vi "nanocal -- nuclear schottky fit V7.vi"() -> ()   [LabVIEW 2021]
uses:
  filename-pattern.ctl
  show-win- control.ctl
  cursor winow.ctl
  nanocal_data_read_format.ctl
  3-lorentzian-parameters.ctl
  nameformattingitem.ctl
  nanocal_side_selector.ctl
  filename-action.ctl
  nanocal -- gradient descent -- parameters.ctl
  3-lorentzian-heat-response action.ctl
  nanocal-goodness-weighting-strategy.ctl
  nanocal generate curvature ellipse -- action.ctl
  3D curvature triplet control.ctl
  3D curvature tensor.ctl
  <vilib>/Analysis/Matrix/Datatypes/RealMatrix.ctl
  <vilib>/Analysis/Matrix/Datatypes/ComplexMatrix.ctl
  cursor window action.ctl
  cursor action.ctl
  2Dwindow.ctl
  publisher action.ctl
  <vilib>/Utility/miscctls.llb/LVMapReplaceAction.ctl
  mathematica string map action.ctl
  nanocal -- gradient descent -- action.ctl
  array action.ctl
  cursor sate.ctl
  nanocal -- defaut parameter manager action-- V1.ctl
  nanocal -- plotstring file action.ctl
  file -- read-write control.ctl
  array -- freq-voltage transformations action.ctl
  nanocal_raw_file_manage_action_V1.ctl
  KM_file -- read-write control.ctl
  replace cursor action stack.vi
  Q -- range multiplier -- real -- V2.vi
  Q - not nan and gtr than zero - Real.vi
  Q - not nan -- real.vi
  Q -- check range -- i -- real.vi
  array - smart min max.vi
  3-lorentzian-heat-response -- V4.vi/142dd4c5-f9ed-c64b-bc14-a88e3e2c450a.vi
  array -- bilinear regression 3D -- curvature wrapper -- V2.vi
  array -- gaussian random.vi
  <vilib>/Analysis/baseanly.llb/Mean.vi
  <vilib>/Analysis/baseanly.llb/Mean (DBL).vi
  <vilib>/AdvancedString/Delimited String to 1D String Array.vi
  array -- freq-voltage transformations.vi/05c44075-957c-bc42-b6fa-2799d0bc0485.vi
  tale of three indices.vi
  filter -- window span logic.vi
  linear interp iiii- complex - z-omega - divide.vi
  linear interpolation iiii- complex.vi
  containing bix.vi
  3D curvature tensor algebra --V2.vi
  array -- bilinear regression 3D -- V3.vi
  <vilib>/Array/Sort 2D Array - Pop Stack.vi
  <vilib>/Array/Sort 2D Array - Push Stack.vi
  array -- freq-voltage transformations.vi/05c44075-957c-bc42-b6fa-2799d0bc0485.vi/269d4b3b-47f5-49e3-8884-44851e4dd9d5.vi
  array -- freq-voltage transformations.vi/05c44075-957c-bc42-b6fa-2799d0bc0485.vi/6d99389c-673d-4efb-bf33-19b32bcf4cf8.vi
  command stack.vi
  tale of three indices -- check state.vi
  Q -- check range -- i -- integer.vi
  linear interp iiii- complex - z-omega.vi
  line -- complex.vi
  <vilib>/Analysis/7linalg.llb/Solve Linear Equations.vi
  <vilib>/Analysis/7linalg.llb/Solve Linear Equations (single right hand).vi
  array -- linear regression 3D -- V2.vi
  <vilib>/Analysis/baseanly.llb/A x B.vi
  <vilib>/Analysis/baseanly.llb/Real A x B.vi
  Q - not nan -- integer.vi
  <vilib>/Analysis/baseanly.llb/Complex A x B.vi
  <vilib>/Analysis/baseanly.llb/Solve Linear Equations By Cholesky.vi
  <vilib>/Analysis/baseanly.llb/Real Matrix to Compact Array.vi
  <vilib>/Analysis/baseanly.llb/Real Compact Tri-Matrix Linear Eqs.vi
  <vilib>/Analysis/Matrix/Numeric/Conversions/Array To Matrix.vi
  <vilib>/Analysis/Matrix/Numeric/Conversions/Array To Matrix - RA2.vi
  <vilib>/Analysis/7linalg.llb/Solve Linear Eqs (General).vi
  <vilib>/Analysis/7linalg.llb/Solve Linear Eqs (Gen, single right hand).vi
  <vilib>/Analysis/Matrix/Numeric/Conversions/Matrix To Array.vi
  <vilib>/Analysis/Matrix/Numeric/Conversions/Matrix To Array - RM.vi
  <vilib>/Analysis/7linalg.llb/Eigenvalues and Vectors.vi
  <vilib>/Analysis/7linalg.llb/Real Eigenvalues and Vectors.vi
  <vilib>/Analysis/baseanly.llb/Inverse Matrix.vi
  <vilib>/Analysis/baseanly.llb/Real Inverse Matrix.vi
  <vilib>/Analysis/polynomials.llb/Polynomial Roots.vi
  <vilib>/Analysis/polynomials.llb/Polynomial Roots (DBL).vi
  <vilib>/Comparison/Less/Less Functor/Less Functor.lvclass
  <vilib>/Analysis/Matrix/NI_Matrix.lvlib
panel:
  in  "tab 8":T1(tab)
  in  "sweeper panel":enum32{"main"}(tab)
  out "Plot: circles":cluster{"Freq out (Hz)":dbl[], dbl[]}[](graph)
  in  "scale gauge: Plot: circles":dbl(slide)=27302460.057190996 min=0.0 max=0.3 step=1e-06 scale=1000000.0..10000000000.0 scale format="%#_3p"
  in  "parameter tab":enum32{"logarithmic derivatives"}(tab)
  in  "factors":cluster{"scaling":dbl, "what":T2}[](array[cluster])=[{"scaling"=1.0, "what"=enum."ζ"}, {"scaling"=1.0, "what"=enum."τ1"}, {"scaling"=1.0, "what"=enum."τS"}, {"scaling"=1.0, "what"=enum."τN"}, {"scaling"=1.0, "what"=enum."τC"}, {"scaling"=1.0, "what"=enum."κ0"}]
  in  "tab77":enum32{"Page 1"}(tab)
  in  "τC":dbl(slide)=0.0015347438601793005 min=0.0 max=0.3 step=1e-06 scale=0.0001..1.0 scale format="%#_3p"
  in  "τN":dbl(slide)=0.020275054268168058 min=0.0 max=0.3 step=1e-06 scale=1e-06..1.0 scale format="%#_3p"
  in  "τS":dbl(slide)=0.018315346057340396 min=0.0 max=0.3 step=1e-06 scale=0.0001..1.0 scale format="%#_3p"
  in  "ζ":dbl(slide)=0.10152887026018578 min=0.0 max=0.3 step=1e-06 scale=1e-05..1.0 scale format="%#_3p"
  in  "T1":dbl(slide)=0.4652876432055127 min=0.0 max=0.3 step=1e-06 scale=0.0001..1.0 scale format="%#_3p"
  in  "κ0":dbl(slide)=1.5437103804183895e-09 min=0.0 max=0.3 step=1e-12 scale=1e-10..1e-06 scale format="%#_3p"
  in  "newton parameters":T3={"newton action"=enum."onlygrads", "weighting"=enum."dω √(|dz/dω|)", "PID-P"=9.612492635866019e-06, "PID-I"=12} {"PID-P" scale=1e-09..1.0 scale format="%#_3p"}
  out "vector v=dlogG/dlogα of logarithmic derivatives":dbl[](array[numeric])=[0.019124578634142967, 0.4891903036062691, -0.015428448808932498, -0.05822768648048974, -0.04691104340908931, 0.018178792884011388] format="%#11.9f"
  in  "tab 4":enum32{"Page 1"}(tab)
  in  "go / pause!":bool
  in  "plots tab":enum32{"Page 1"}(tab)
  in  "X selector":T2=enum."T (K)"
  out "Plot:  colors":cluster{"Freq out (Hz)":dbl[], dbl[]}[](graph)=[{"Freq out (Hz)"=[0.12, 0.148, 0.15, 0.17, 0.2, 0.25, 0.3, 0.36, 0.42, 0.52, 0.62, 0.82, 1.12, 1.7, 1.9, 3.1, 5.7], [0.62728998582, 0.2730109012575849, 0.4360358231158382, 0.31273882707493267, 0.21185679953244455, 0.14497429295634315, 0.10320507255338958, 0.06738649827292763, 0.022507492936216303, 0.021849716434935364, 0.021729475893381252, 0.0198519726342436, 0.016283381951146165, 0.01886089700009046, 0.017534515105553365, 0.01657901647493233, 0.017491792324152208]}, {"Freq out (Hz)"=[0.12, 0.148, 0.15, 0.17, 0.2, 0.25, 0.3, 0.36, 0.42, 0.52, 0.62, 0.82, 1.12, 1.7, 1.9, 3.1, 5.7], [0.23974349678, 0.07091543775458298, 0.13629832485566626, 0.15316677568416495, 0.17371303124805412, 0.27815367910908206, 0.4568771678095196, 0.03375938315839582, 0.03387143424300576, 0.033883152649051125, 0.03390178634313435, 0.03384656153160249, 0.03390452446017073, 0.03378369231014688, 0.02323861783817173, 0.029207680038740087, 0.02587551529326107]}, {"Freq out (Hz)"=[0.12, 0.148, 0.15, 0.17, 0.2, 0.25, 0.3, 0.36, 0.42, 0.52, 0.62, 0.82, 1.12, 1.7, 1.9, 3.1, 5.7], [0.076926495749, 0.13557684408337248, 0.03542880244691447, 0.02942840377205427, 0.02504707721851352, 0.020087180736490247, 0.018190810679879554, 0.0163524675075112, 0.016835987172777216, 0.01819702773822382, 0.020153498516221252, 0.023547995635674095, 0.031661688913314306, 0.03349591654527996, 0.014265591932458873, 0.009191722708188048, 0.005854448603805341]}, {"Freq out (Hz)"=[0.12, 0.148, 0.15, 0.17, 0.2, 0.25, 0.3, 0.36, 0.42, 0.52, 0.62, 0.82, 1.12, 1.7, 1.9, 3.1, 5.7], [0.159415903746, 0.04012911681217574, 0.042141009445427945, 0.032059842594624494, 0.02279985029361622, 0.018878235168909133, 0.020353539568818982, 5.5602042137039274e-05, 0.00021346840235837033, 0.00021340250099372794, 0.00021321792059620005, 0.00027413175252649695, 0.0002745370162211529, 0.0004261574975821111, 0.000383027800546881, 0.0002822141564676873, 0.00033678261197217014]}, {"Freq out (Hz)"=[0.12, 0.148, 0.15, 0.17, 0.2, 0.25, 0.3, 0.36, 0.42, 0.52, 0.62, 0.82, 1.12, 1.7, 1.9, 3.1, 5.7], [0.000763641667, 0.0009923872987074498, 0.0008634344957269274, 0.000966119229084584, 0.0011194877919145127, 0.0013606502621125451, 0.0015326336783234693, 0.002052818741953473, 0.0017781658353584764, 0.001801850307392029, 0.0018089734240976446, 0.002984103948241005, 0.003250738484609814, 0.0031602960429135524, 0.002949269667352954, 0.002421267656945163, 0.002022629565026247]}]
  in  "tab 55":enum32{"main", "more", "file", "notes"}(tab)
  in  "gradient descent monitor tab":enum32{"Page 2"}(tab)
  out "|dln G/dln α_i |":dbl(slide)=56.37329977448589 scale=0.001..1.0 scale format="%#_3p"
  out "Goodness":dbl(slide)=0.00019249505739334056 scale=0.001..1.0 scale format="%#_3p"
  in  "update rate":i32=1000
  in  "total # steps":i32=50000
  out "|v_i| = | dlogG/dlogα_i | (log scale slider)":dbl[](array[slide])=[0.019124578634142967, 0.4891903036062691, 0.015428448808932498, 0.05822768648048974, 0.04691104340908931, 0.018178792884011388] scale=1e-08..10.0 scale format="%#_2p"
  in  "oscillations & stuff tab":enum32{"Page 2", "Page 3"}(tab)
  in  "tab 9":enum32{"Page 1"}(tab)
  in  "#grad steps":i32=400
  out "Plot: oscillations":cluster{"Array":i32[], "Array":dbl[]}(graph)={"Array"=[0, 1, 2, 3, 4, 5, 6, 7, 8, 9, 10, 11, 12, 13, 14, 15, 16, 17, 18, 19, 20, 21, 22, 23, 24, 25, 26, 27, 28, 29, 30, 31, 32, 33, 34, 35, 36, 37, 38, 39, 40, 41, 42, 43, 44, 45, 46, 47, 48, 49, 50, 51, 52, 53, 54, 55, 56, 57, 58, 59, 60, 61, 62, 63, 64, 65, 66, 67, 68, 69, 70, 71, 72, 73, 74, 75, 76, 77, 78, 79, 80, 81, 82, 83, 84, 85, 86, 87, 88, 89, 90, 91, 92, 93, 94, 95, 96, 97, 98, 99, 100, 101, 102, 103, 104, 105, 106, 107, 108, 109, 110, 111, 112, 113, 114, 115, 116, 117, 118, 119, 120, 121, 122, 123, 124, 125, 126, 127, 128, 129, 130, 131, 132, 133, 134, 135, 136, 137, 138, 139, 140, 141, 142, 143, 144, 145, 146, 147, 148, 149, 150, 151, 152, 153, 154, 155, 156, 157, 158, 159, 160, 161, 162, 163, 164, 165, 166, 167, 168, 169, 170, 171, 172, 173, 174, 175, 176, 177, 178, 179, 180, 181, 182, 183, 184, 185, 186, 187, 188, 189, 190, 191, 192, 193, 194, 195, 196, 197, 198, 199, 200, 201, 202, 203, 204, 205, 206, 207, 208, 209, 210, 211, 212, 213, 214, 215, 216, 217, 218, 219, 220, 221, 222, 223, 224, 225, 226, 227, 228, 229, 230, 231, 232, 233, 234, 235, 236, 237, 238, 239, 240, 241, 242, 243, 244, 245, 246, 247, 248, 249, 250, 251, 252, 253, 254, 255, 256, 257, 258, 259, 260, 261, 262, 263, 264, 265, 266, 267, 268, 269, 270, 271, 272, 273, 274, 275, 276, 277, 278, 279, 280, 281, 282, 283, 284, 285, 286, 287, 288, 289, 290, 291, 292, 293, 294, 295, 296, 297, 298, 299, 300, 301, 302, 303, 304, 305, 306, 307, 308, 309, 310, 311, 312, 313, 314, 315, 316, 317, 318, 319, 320, 321, 322, 323, 324, 325, 326, 327, 328, 329, 330, 331, 332, 333, 334, 335, 336, 337, 338, 339, 340, 341, 342, 343, 344, 345, 346, 347, 348, 349, 350, 351, 352, 353, 354, 355, 356, 357, 358, 359, 360, 361, 362, 363, 364, 365, 366, 367, 368, 369, 370, 371, 372, 373, 374, 375, 376, 377, 378, 379, 380, 381, 382, 383, 384, 385, 386, 387, 388, 389, 390, 391, 392, 393, 394, 395, 396, 397, 398, 399], "Array"=[1.602606484205158e-10, 1.5784530103877918e-10, 1.554421775757514e-10, 1.5305127610697362e-10, 1.50672596713761e-10, 1.4830613717349908e-10, 1.4595189851617993e-10, 1.4360987835655876e-10, 1.4128007693858108e-10, 1.3896249247331328e-10, 1.366571244728644e-10, 1.3436397375038607e-10, 1.3208303678222122e-10, 1.2981431527598827e-10, 1.2755780643986664e-10, 1.2531351038227653e-10, 1.2308142688637752e-10, 1.2086155389218547e-10, 1.1865389137259534e-10, 1.1645843870419087e-10, 1.1427519523645076e-10, 1.1210415896360099e-10, 1.0994533143062965e-10, 1.0779870957466561e-10, 1.0566429301623811e-10, 1.0354208224323813e-10, 1.0143207495173605e-10, 9.933427143988746e-11, 9.724867078612053e-11, 9.517527174360274e-11, 9.311407274024096e-11, 9.106507570049403e-11, 8.902827753438577e-11, 8.700367854007178e-11, 8.499127760624482e-11, 8.299107321502186e-11, 8.100306582718882e-11, 7.902725476511933e-11, 7.706363748093831e-11, 7.511221524858329e-11, 7.317298530333874e-11, 7.124594973229384e-11, 6.933110642125435e-11, 6.74284519820885e-11, 6.55379904805544e-11, 6.365971733589791e-11, 6.179363292758977e-11, 5.99397377164159e-11, 5.809802901897594e-11, 5.62685072960558e-11, 5.445117121950782e-11, 5.2646021304328036e-11, 5.085305375580884e-11, 4.90722720976073e-11, 4.7303672887381507e-11, 4.554725501382424e-11, 4.380301939850735e-11, 4.2070964794598334e-11, 4.0351089955264693e-11, 3.864339363367393e-11, 3.6947876453242295e-11, 3.526453529688854e-11, 3.359337469115674e-11, 3.193438775136309e-11, 3.0287577648798955e-11, 2.8652942594530745e-11, 2.703048039304906e-11, 2.5420191342509502e-11, 2.3822075497122175e-11, 2.223613228768094e-11, 2.06623592205208e-11, 1.910075737984393e-11, 1.7551325329082448e-11, 1.6014061685878586e-11, 1.4488966911018267e-11, 1.2976039405303286e-11, 1.1475278301371905e-11, 9.986684249745428e-12, 8.510254865179076e-12, 7.045989171890893e-12, 5.593888741974029e-12, 4.153951678074683e-12, 2.726176543624975e-12, 1.310563718095667e-12, -9.288921086307578e-14, -1.4841796953761477e-12, -2.8633126685634336e-12, -4.230285284394231e-12, -5.5851015002064686e-12, -6.927759283121074e-12, -8.25825985286549e-12, -9.576604646007597e-12, -1.0882793255971579e-11, -1.2176828799838682e-11, -1.3458708648418638e-11, -1.4728437138520137e-11, -1.5986011993318616e-11, -1.7231435923319507e-11, -1.8464707058274063e-11, -1.968582908446967e-11, -2.0894800999019317e-11, -2.209162483480208e-11, -2.3276299155250077e-11, -2.4448826887709177e-11, -2.560920716481764e-11, -2.6757440393151283e-11, -2.7893529933736838e-11, -2.901747386211545e-11, -3.012927385880049e-11, -3.1228928893799884e-11, -3.231644387312847e-11, -3.339181557128479e-11, -3.445504490984068e-11, -3.550613473482685e-11, -3.654508477519275e-11, -3.7571895356199037e-11, -3.8586568022833806e-11, -3.95891017993151e-11, -4.057949917930792e-11, -4.1557760054392046e-11, -4.252388499377362e-11, -4.3477875135864916e-11, -4.4419729748829476e-11, -4.534945205816876e-11, -4.626704019363402e-11, -4.717249700125596e-11, -4.8065821125781866e-11, -4.8947015196402e-11, -4.981607826443947e-11, -5.06730123898784e-11, -5.1517817654033946e-11, -5.235049438216677e-11, -5.3171043468743656e-11, -5.397946564560108e-11, -5.4775762945618103e-11, -5.555993173671746e-11, -5.633197817174647e-11, -5.709189975704014e-11, -5.783969784785119e-11, -5.857537347417167e-11, -5.929892650047633e-11, -6.001035749597129e-11, -6.070966803274971e-11, -6.139685976421991e-11, -6.207193025092698e-11, -6.273488347731393e-11, -6.338571738339661e-11, -6.402443448994509e-11, -6.465103563721604e-11, -6.526551906338093e-11, -6.586788788552102e-11, -6.645814234758178e-11, -6.703628272061377e-11, -6.760230924856246e-11, -6.815622225668852e-11, -6.869802364234574e-11, -6.92277144355262e-11, -6.974529431096922e-11, -7.02507637023557e-11, -7.074412377520295e-11, -7.122537425846044e-11, -7.169451759158306e-11, -7.215155358483542e-11, -7.259648229242764e-11, -7.302930525934781e-11, -7.345002235007066e-11, -7.385863573300053e-11, -7.425514394446449e-11, -7.463954836682031e-11, -7.501184951506402e-11, -7.537205018101623e-11, -7.572014854863827e-11, -7.605614570213234e-11, -7.638004324069664e-11, -7.669184132696148e-11, -7.699154020487237e-11, -7.727914093152641e-11, -7.755464391349942e-11, -7.78180500452582e-11, -7.806935818839046e-11, -7.830857354706663e-11, -7.853569248920944e-11, -7.875071693927774e-11, -7.895364817120908e-11, -7.914448623921357e-11, -7.932323081803055e-11, -7.948988564815754e-11, -7.964444780224865e-11, -7.978691999080932e-11, -7.991730213252439e-11, -8.003559487791516e-11, -8.014180044959608e-11, -8.023591646232238e-11, -8.031794657527638e-11, -8.038788943320538e-11, -8.044574601189132e-11, -8.04915181544779e-11, -8.05252047496579e-11, -8.054680820978113e-11, -8.055632696275447e-11, -8.055376434249958e-11, -8.053911874981827e-11, -8.051239194653906e-11, -8.04735845560782e-11, -8.042269622606998e-11, -8.035972858281767e-11, -8.028468235815774e-11, -8.019755785024577e-11, -8.009835560118285e-11, -7.998707509597296e-11, -7.986372002090347e-11, -7.972828809914984e-11, -7.95807809028052e-11, -7.942120070869411e-11, -7.924954545683247e-11, -7.906581574353144e-11, -7.887001520086832e-11, -7.866214087439219e-11, -7.844219772432798e-11, -7.821018173912765e-11, -7.796609717428474e-11, -7.770994202402522e-11, -7.744171880911914e-11, -7.716142739404123e-11, -7.686906783300161e-11, -7.656464180651364e-11, -7.624814833879535e-11, -7.591959041140274e-11, -7.557896696723868e-11, -7.522627854840425e-11, -7.486152688962293e-11, -7.448471161142396e-11, -7.40958333372236e-11, -7.369489445226661e-11, -7.328189311340931e-11, -7.285683116379539e-11, -7.241971009420284e-11, -7.197052830543345e-11, -7.150928845378254e-11, -7.103598988872882e-11, -7.055063353184413e-11, -7.005321981680933e-11, -6.954375115597426e-11, -6.902222632961148e-11, -6.848864482272496e-11, -6.794301021318186e-11, -6.738532046810311e-11, -6.68155786774649e-11, -6.623378291680838e-11, -6.563993576111371e-11, -6.503403691222528e-11, -6.441608715618968e-11, -6.378608798378489e-11, -6.314403874448961e-11, -6.248993911304318e-11, -6.182379337204419e-11, -6.114559734731427e-11, -6.045535664959967e-11, -5.975306756550794e-11, -5.903873283264957e-11, -5.831235356233179e-11, -5.7573928372196825e-11, -5.682345953906924e-11, -5.606094722557936e-11, -5.5286391919618164e-11, -5.44997939464463e-11, -5.3701154769736706e-11, -5.289047322397204e-11, -5.2067752290708286e-11, -5.123299126521402e-11, -5.038619177379251e-11, -4.9527352867766855e-11, -4.8656474845292647e-11, -4.777355960372369e-11, -4.6878609040413785e-11, -4.597161998407158e-11, -4.5052597665972555e-11, -4.4121538020358564e-11, -4.317844546535346e-11, -4.222331826623377e-11, -4.125615745299155e-11, -4.027696354062284e-11, -3.928573888726736e-11, -3.828248259845832e-11, -3.726719502656142e-11, -3.623987665946765e-11, -3.520052871690445e-11, -3.414915171386784e-11, -3.308574705982066e-11, -3.2010313562140513e-11, -3.092285273871044e-11, -2.982336594478316e-11, -2.871185255694242e-11, -2.7588313442549958e-11, -2.6452750038173656e-11, -2.5305161340926502e-11, -2.414554913974208e-11, -2.297391384119621e-11, -2.1790256637911273e-11, -2.0594575659638528e-11, -1.9386874484245142e-11, -1.8167153220151333e-11, -1.6935410756049873e-11, -1.569164926034511e-11, -1.4435867459099486e-11, -1.3168069553596423e-11, -1.1888251315447448e-11, -1.0596416783305654e-11, -9.292566011381148e-12, -7.976699487564909e-12, -6.6488159379193834e-12, -5.3089191571521754e-12, -3.957007220804429e-12, -2.5930814570238048e-12, -1.2171420826507379e-12, 1.7080892364580713e-13, 1.5707728900134915e-12, 2.982747539627753e-12, 4.406732953803755e-12, 5.842729945693126e-12, 7.290735100059023e-12, 8.750749202948022e-12, 1.0222772254360121e-11, 1.1706803874824562e-11, 1.3202842438038084e-11, 1.4710886453222702e-11, 1.623093808878276e-11, 1.776299498657853e-11, 1.930705728213529e-11, 2.0863122400472875e-11, 2.2431192862361338e-11, 2.401126641808117e-11, 2.560334192922009e-11, 2.7207420181824676e-11, 2.8823499549591666e-11, 3.045157997831095e-11, 3.2091660709041014e-11, 3.3743741389416146e-11, 3.540782185680602e-11, 3.708389991570124e-11, 3.8771977083984846e-11, 4.047205078667668e-11, 4.218412199955869e-11, 4.390818950290344e-11, 4.564425335092104e-11, 4.7392310236794855e-11, 4.915236406365271e-11, 5.092441044047581e-11, 5.270845140014323e-11, 5.4504485722927515e-11, 5.631251069832324e-11, 5.813252732921742e-11, 5.996453756717396e-11, 6.18085360453921e-11, 6.366452509490653e-11, 6.553250376704033e-11, 6.74124723599491e-11, 6.930442759392128e-11, 7.120837207104207e-11, 7.31243031079111e-11, 7.505222097557891e-11, 7.699212393932203e-11, 7.894401362544372e-11, 8.090788729633348e-11, 8.288374595487834e-11, 8.48715881645104e-11, 8.687141330181343e-11, 8.888322109573688e-11, 9.090701219680204e-11, 9.294278403002877e-11, 9.499053635147157e-11, 9.7050269432181e-11, 9.912198254032056e-11, 1.0120567421221735e-10, 1.0330134515260277e-10, 1.0540899416885442e-10, 1.0752862134228748e-10, 1.0966022496528352e-10, 1.1180380444153135e-10, 1.1395936147864938e-10, 1.1612689087246719e-10, 1.1830639790847038e-10, 1.2049787841248057e-10, 1.2270133284528369e-10, 1.249167597974169e-10, 1.2714415837441345e-10, 1.2938353104283325e-10, 1.3163487230035027e-10, 1.3389818778481583e-10, 1.3617347074707138e-10, 1.3846072511734982e-10, 1.407599478869901e-10, 1.4307113935414784e-10, 1.4539429903093204e-10, 1.4772942613129614e-10, 1.5007651962524807e-10, 1.5243558027172935e-10, 1.5480660625470134e-10, 1.5718959873968139e-10, 1.5958455485353372e-10]}
  out "current step ind":i32=926
  out "current  ind":i32=1
  out "correct temperature":dbl=1040.0 min=10.0 max=10000.0 step=10.0
  in  "generate empty string from filelist !":bool
  in  "toggle generate labview files":bool
  in  "data file formatting":T6=enum."raw nanocal"
  in  "save data":enum32{"save/read"}(tab)
  in  "Save to file :s":bool
  in  "Freq sweep name template":T7={"prefix"="RuCl3-rod", "group"="f"}
  in  "Save folder":path=path "/opt/data"
  in  "freq sweep file name":string="f013_RuCl3-rod_082821.dat"
  in  "side":T8=enum."ref"
  in  "string notes":string="\"T\"-> 0.225000,    \"ζ\"-> 0.006057  , \"τ1\"-> 0.011106  , \"τS\"-> 0.134857  , \"τN\"-> 0.000042  , \"τC\"-> 0.012982  , \"κ0\"-> 0.000000101776  , \"mm1\"-> 0.000071  , \"mm2\"-> 0.148631  , \"mm3\"-> 0.011103 "
  in  "load! :l":bool
  in  "Read from file":path=path "/opt/new/Dropbox/shared_AkashAndreas/paper-CeCoIn5/Original RAW data/Original RAW files (IDS0396 to IDS0xxx)/IDS0446_220528_RAW_cal_CeCoIn5_5th_051_6T_0deg__fSweep_0.30K_raw_.dat"
  in  "parse! :p":bool
  in  "String":string=" <|    \"ζ\" -> 0.101528870260   ,  \"τ1\" -> 0.465287643206   ,  \"τS\" -> 0.018315346057   ,  \"τN\" -> 0.020275054268   ,  \"τC\" -> 0.001534743860   ,  \"κ0\" -> 0.000000001544   ,  \"mm1\" -> 0.000132261454   ,  \"mm2\" -> 0.020546066419   ,  \"mm3\" -> 0.488652499266   ,  \"T\" -> 0.300000000000   ,  \"B\" -> 6.000000000000   ,  \"θ\" -> 0.000000000000   ,  \"Reoff\" -> 0.000000000000   ,  \"Imoff\" -> 0.000000000000   ,  \"στ1\" -> 0.000000000000   ,  \"στS\" -> 0.000000000000   ,  \"στN\" -> 0.000000000000    |> "
  in  "newton is active":bool
  out "file IDS":string="IDS0446_220528_RAW_cal_"
  out "notes":string="------------\n\n/opt/new/Dropbox/desktop_data/Indium-nanocal-cell12-June2021/labview-ready-files\nIndium_June2021_*_ark.dat\n\n---------------------\n/opt/new/Dropbox/shared_AkashAndreas/paper-CeCoIn5/labviewreadydata\nCeCoIn5_*_labview_.dat\n--------------------------------\n\n  48 ->   <| \"ζ\"->  0.219100303741  , \"τ1\"-> 0.028643012604  , \"τS\"-> 0.279362928811  , \"τN\"-> 0.246156444058  , \"τC\"-> 0.001272401549  , \"κ0\"-> 0.000000000760  , \"mm1\"-> 0.000227975653  , \"mm2\"-> 0.014929571562  , \"mm3\"-> 0.655418694024  , \"T\"->  0.148000000000  , \"B\"-> 12.000000000000  , \"θ\"-> 0.000000000000  |>   , \r49 ->   <| \"ζ\"->  0.172530402516  , \"τ1\"-> 0.028151242536  , \"τS\"-> 0.147833386881  , \"τN\"-> 0.151615465647  , \"τC\"-> 0.001078987959  , \"κ0\"-> 0.000000001040  , \"mm1\"-> 0.000157922197  , \"mm2\"-> 0.013374167913  , \"mm3\"-> 0.366811023972  , \"T\"->  0.179000000000  , \"B\"-> 12.000000000000  , \"θ\"-> 0.000000000000  |>   , \r50 ->   <| \"ζ\"->  0.133463068512  , \"τ1\"-> 0.025720252342  , \"τS\"-> 0.123146502099  , \"τN\"-> 0.097478248186  , \"τC\"-> 0.001335222055  , \"κ0\"-> 0.000000001204  , \"mm1\"-> 0.000155896243  , \"mm2\"-> 0.013755191011  , \"mm3\"-> 0.263214393590  , \"T\"->  0.197000000000  , \"B\"-> 12.000000000000  , \"θ\"-> 0.000000000000  |>   , \r51 ->   <| \"ζ\"->  0.081993362741  , \"τ1\"-> 0.028064095915  , \"τS\"-> 0.091433392476  , \"τN\"-> 0.030443971714  , \"τC\"-> 0.001450504959  , \"κ0\"-> 0.000000001536  , \"mm1\"-> 0.000108446090  , \"mm2\"-> 0.019905820843  , \"mm3\"-> 0.141370833064  , \"T\"->  0.250000000000  , \"B\"-> 12.000000000000  , \"θ\"-> 0.000000000000  |>   , \r52 ->   <| \"ζ\"->  0.054088186012  , \"τ1\"-> 0.023838802615  , \"τS\"-> 0.069079396629  , \"τN\"-> 0.016435267456  , \"τC\"-> 0.002025071743  , \"κ0\"-> 0.000000001955  , \"mm1\"-> 0.000101234646  , \"mm2\"-> 0.018244822177  , \"mm3\"-> 0.097657814678  , \"T\"->  0.300000000000  , \"B\"-> 12.000000000000  , \"θ\"-> 0.000000000000  |>   , \r53 ->   <| \"ζ\"->  0.039314966212  , \"τ1\"-> 0.020712803909  , \"τS\"-> 0.055413767550  , \"τN\"-> 0.008474403424  , \"τC\"-> 0.002674063387  , \"κ0\"-> 0.000000002415  , \"mm1\"-> 0.000096818147  , \"mm2\"-> 0.017190811405  , \"mm3\"-> 0.072499170001  , \"T\"->  0.360000000000  , \"B\"-> 12.000000000000  , \"θ\"-> 0.000000000000  |>   , \r54 ->   <| \"ζ\"->  0.031945976845  , \"τ1\"-> 0.019000922826  , \"τS\"-> 0.045624146388  , \"τN\"-> 0.005314716063  , \"τC\"-> 0.002488383471  , \"κ0\"-> 0.000000002954  , \"mm1\"-> 0.000073272643  , \"mm2\"-> 0.016306894362  , \"mm3\"-> 0.057675293464  , \"T\"->  0.430000000000  , \"B\"-> 12.000000000000  , \"θ\"-> 0.000000000000  |>   , \r55 ->   <| \"ζ\"->  0.023031239946  , \"τ1\"-> 0.018268814012  , \"τS\"-> 0.037269400776  , \"τN\"-> 0.002696792890  , \"τC\"-> 0.003257395394  , \"κ0\"-> 0.000000003720  , \"mm1\"-> 0.000067670174  , \"mm2\"-> 0.016445281937  , \"mm3\"-> 0.045899921957  , \"T\"->  0.512000000000  , \"B\"-> 12.000000000000  , \"θ\"-> 0.000000000000  |>   , \r56 ->   <| \"ζ\"->  0.019920170845  , \"τ1\"-> 0.016368892412  , \"τS\"-> 0.030579536580  , \"τN\"-> 0.001736017565  , \"τC\"-> 0.004971418152  , \"κ0\"-> 0.000000004410  , \"mm1\"-> 0.000083939556  , \"mm2\"-> 0.015095997595  , \"mm3\"-> 0.039119658918  , \"T\"->  0.610000000000  , \"B\"-> 12.000000000000  , \"θ\"-> 0.000000000000  |>   , \r57 ->   <| \"ζ\"->  0.017558473054  , \"τ1\"-> 0.014545104284  , \"τS\"-> 0.022979681288  , \"τN\"-> 0.000840829385  , \"τC\"-> 0.005228030240  , \"κ0\"-> 0.000000006068  , \"mm1\"-> 0.000073916527  , \"mm2\"-> 0.013750428362  , \"mm3\"-> 0.030187552103  , \"T\"->  0.810000000000  , \"B\"-> 12.000000000000  , \"θ\"-> 0.000000000000  |>   , \r58 ->   <| \"ζ\"->  0.011916480594  , \"τ1\"-> 0.012551282481  , \"τS\"-> 0.018233218660  , \"τN\"-> 0.000345702746  , \"τC\"-> 0.004699451527  , \"κ0\"-> 0.000000008451  , \"mm1\"-> 0.000044190864  , \"mm2\"-> 0.012162820727  , \"mm3\"-> 0.023844039179  , \"T\"->  1.120000000000  , \"B\"-> 12.000000000000  , \"θ\"-> 0.000000000000  |>   , \r59 ->   <| \"ζ\"->  0.012831327568  , \"τ1\"-> 0.013315909415  , \"τS\"-> 0.012590836847  , \"τN\"-> 0.000065003013  , \"τC\"-> 0.005276356243  , \"κ0\"-> 0.000000013610  , \"mm1\"-> 0.000047406274  , \"mm2\"-> 0.013137605540  , \"mm3\"-> 0.018225484932  , \"T\"->  1.800000000000  , \"B\"-> 12.000000000000  , \"θ\"-> 0.000000000000  |>   , \r60 ->   <| \"ζ\"->  0.019774146838  , \"τ1\"-> 0.013257273421  , \"τS\"-> 0.007064131508  , \"τN\"-> 0.000028000819  , \"τC\"-> 0.006942241845  , \"κ0\"-> 0.000000023477  , \"mm1\"-> 0.000068886863  , \"mm2\"-> 0.012935419574  , \"mm3\"-> 0.014427582022  , \"T\"->  3.000000000000  , \"B\"-> 12.000000000000  , \"θ\"-> 0.000000000000  |>   , \r61 ->   <| \"ζ\"->  0.029251354442  , \"τ1\"-> 0.014634751206  , \"τS\"-> 0.003873958746  , \"τN\"-> 0.000007000487  , \"τC\"-> 0.006827504775  , \"κ0\"-> 0.000000056438  , \"mm1\"-> 0.000072018576  , \"mm2\"-> 0.010723236476  , \"mm3\"-> 0.014661483476  , \"T\"->  5.500000000000  , \"B\"-> 12.000000000000  , \"θ\"-> 0.000000000000  |>   , \r70 ->   <| \"ζ\"->  0.166131699293  , \"τ1\"-> 0.072775930308  , \"τS\"-> 0.042465819987  , \"τN\"-> 0.161702990281  , \"τC\"-> 0.001278548133  , \"κ0\"-> 0.000000001029  , \"mm1\"-> 0.000178150965  , \"mm2\"-> 0.012296129795  , \"mm3\"-> 0.299667919341  , \"T\"->  0.179000000000  , \"B\"-> 12.000000000000  , \"θ\"-> 90.000000000000  |>   , \r71 ->   <| \"ζ\"->  0.300863384227  , \"τ1\"-> 0.104924004009  , \"τS\"-> 0.071070599729  , \"τN\"-> 0.992887187112  , \"τC\"-> 0.001721587800  , \"κ0\"-> 0.000000000548  , \"mm1\"-> 0.000392216822  , \"mm2\"-> 0.006637384427  , \"mm3\"-> 1.483679717825  , \"T\"->  0.120000000000  , \"B\"-> 12.000000000000  , \"θ\"-> 90.000000000000  |>   , \r72 ->   <| \"ζ\"->  0.222191124978  , \"τ1\"-> 0.096157808510  , \"τS\"-> 0.068016409177  , \"τN\"-> 0.365932480375  , \"τC\"-> 0.001342124138  , \"κ0\"-> 0.000000000769  , \"mm1\"-> 0.000240761160  , \"mm2\"-> 0.013184061080  , \"mm3\"-> 0.614443591912  , \"T\"->  0.148000000000  , \"B\"-> 12.000000000000  , \"θ\"-> 90.000000000000  |>   , \r73 ->   <| \"ζ\"->  0.136299067728  , \"τ1\"-> 0.070555788073  , \"τS\"-> 0.041728112583  , \"τN\"-> 0.122673380524  , \"τC\"-> 0.001576035942  , \"κ0\"-> 0.000000001215  , \"mm1\"-> 0.000183611814  , \"mm2\"-> 0.014077355758  , \"mm3\"-> 0.244680119794  , \"T\"->  0.197000000000  , \"B\"-> 12.000000000000  , \"θ\"-> 90.000000000000  |>   , \r74 ->   <| \"ζ\"->  0.083818989463  , \"τ1\"-> 0.054019568165  , \"τS\"-> 0.033709166928  , \"τN\"-> 0.048192327645  , \"τC\"-> 0.001574712191  , \"κ0\"-> 0.000000001532  , \"mm1\"-> 0.000117096712  , \"mm2\"-> 0.016005996433  , \"mm3\"-> 0.128237582295  , \"T\"->  0.249000000000  , \"B\"-> 12.000000000000  , \"θ\"-> 90.000000000000  |>   , \r75 ->   <| \"ζ\"->  0.057938569833  , \"τ1\"-> 0.045244527663  , \"τS\"-> 0.029709028064  , \"τN\"-> 0.023577376257  , \"τC\"-> 0.002006607539  , \"κ0\"-> 0.000000001948  , \"mm1\"-> 0.000103608352  , \"mm2\"-> 0.017542867394  , \"mm3\"-> 0.085978401835  , \"T\"->  0.300000000000  , \"B\"-> 12.000000000000  , \"θ\"-> 90.000000000000  |>   , \r76 ->   <| \"ζ\"->  0.044154556051  , \"τ1\"-> 0.038823125235  , \"τS\"-> 0.027069314930  , \"τN\"-> 0.013601990730  , \"τC\"-> 0.002287979276  , \"κ0\"-> 0.000000002359  , \"mm1\"-> 0.000089763345  , \"mm2\"-> 0.018083678254  , \"mm3\"-> 0.065404792018  , \"T\"->  0.360000000000  , \"B\"-> 12.000000000000  , \"θ\"-> 90.000000000000  |>   , \r77 ->   <| \"ζ\"->  0.032748569996  , \"τ1\"-> 0.031072007290  , \"τS\"-> 0.024343937548  , \"τN\"-> 0.006961654481  , \"τC\"-> 0.002967111565  , \"κ0\"-> 0.000000002964  , \"mm1\"-> 0.000084402249  , \"mm2\"-> 0.018055855929  , \"mm3\"-> 0.048229666078  , \"T\"->  0.430000000000  , \"B\"-> 12.000000000000  , \"θ\"-> 90.000000000000  |>   , \r78 ->   <| \"ζ\"->  0.027599263457  , \"τ1\"-> 0.026239105728  , \"τS\"-> 0.022370859308  , \"τN\"-> 0.003857632966  , \"τC\"-> 0.003499360499  , \"κ0\"-> 0.000000003681  , \"mm1\"-> 0.000081816106  , \"mm2\"-> 0.017901054668  , \"mm3\"-> 0.038707974796  , \"T\"->  0.512000000000  , \"B\"-> 12.000000000000  , \"θ\"-> 90.000000000000  |>   , \r79 ->   <| \"ζ\"->  0.020568815513  , \"τ1\"-> 0.023045965648  , \"τS\"-> 0.020791387386  , \"τN\"-> 0.002229171297  , \"τC\"-> 0.004427475438  , \"κ0\"-> 0.000000004398  , \"mm1\"-> 0.000074037290  , \"mm2\"-> 0.017820522459  , \"mm3\"-> 0.033072945644  , \"T\"->  0.610000000000  , \"B\"-> 12.000000000000  , \"θ\"-> 90.000000000000  |>   , \r80 ->   <| \"ζ\"->  0.016159836955  , \"τ1\"-> 0.019958638777  , \"τS\"-> 0.018730096307  , \"τN\"-> 0.000899236968  , \"τC\"-> 0.005152267403  , \"κ0\"-> 0.000000006087  , \"mm1\"-> 0.000064651231  , \"mm2\"-> 0.017530317649  , \"mm3\"-> 0.027462477400  , \"T\"->  0.810000000000  , \"B\"-> 12.000000000000  , \"θ\"-> 90.000000000000  |>   , \r81 ->   <| \"ζ\"->  0.014495870556  , \"τ1\"-> 0.019990087457  , \"τS\"-> 0.016832201384  , \"τN\"-> 0.000455517238  , \"τC\"-> 0.005555782498  , \"κ0\"-> 0.000000008420  , \"mm1\"-> 0.000060055560  , \"mm2\"-> 0.018114231010  , \"mm3\"-> 0.024909902538  , \"T\"->  1.100000000000  , \"B\"-> 12.000000000000  , \"θ\"-> 90.000000000000  |>   , \r82 ->   <| \"ζ\"->  0.014043763709  , \"τ1\"-> 0.018292068543  , \"τS\"-> 0.011311396743  , \"τN\"-> 0.000128802259  , \"τC\"-> 0.008087849636  , \"κ0\"-> 0.000000014258  , \"mm1\"-> 0.000065912054  , \"mm2\"-> 0.017276417784  , \"mm3\"-> 0.020638450794  , \"T\"->  1.800000000000  , \"B\"-> 12.000000000000  , \"θ\"-> 90.000000000000  |>   , \r83 ->   <| \"ζ\"->  0.016187684631  , \"τ1\"-> 0.018325345271  , \"τS\"-> 0.007510087776  , \"τN\"-> 0.000028419157  , \"τC\"-> 0.008115463080  , \"κ0\"-> 0.000000024747  , \"mm1\"-> 0.000062903858  , \"mm2\"-> 0.015524812312  , \"mm3\"-> 0.018513630087  , \"T\"->  3.000000000000  , \"B\"-> 12.000000000000  , \"θ\"-> 90.000000000000  |>   , \r84 ->   <| \"ζ\"->  0.027897403691  , \"τ1\"-> 0.014639690770  , \"τS\"-> 0.004105291179  , \"τN\"-> 0.000006999171  , \"τC\"-> 0.007414449545  , \"κ0\"-> 0.000000059701  , \"mm1\"-> 0.000073450671  , \"mm2\"-> 0.011534391407  , \"mm3\"-> 0.014673310811  , \"T\"->  5.700000000000  , \"B\"-> 12.000000000000  , \"θ\"-> 90.000000000000  |>   , \r"
  in  "backup string :b":string=" <| \"ζ\"->  0.167234158379  , \"τ1\"-> 0.020665214756  , \"τS\"-> 0.072250691270  , \"τN\"-> 0.020708769022  , \"τC\"-> 0.001243822553  , \"κ0\"-> 0.000000001059  , \"mm1\"-> 0.000000000000  , \"mm2\"-> 0.000000000000  , \"mm3\"-> 0.000000000000  , \"T\"->  5.700000000000  , \"B\"-> 12.000000000000  , \"θ\"-> 45.000000000000  |> "
  in  "tab 7":enum32{"Page 1"}(tab)
  in  "tab 3":enum32{"Page 1"}(tab)
  out "key":string="IDS0446_220528_RAW_cal__ref_"
  out "T (K)":dbl=0.3 format="%#_10f"
  out "θ (deg)":dbl format="%#_10f"
  out "B (T)":dbl=6.0
  in  "tab 6":enum32{"Page 1"}(tab)
  in  "τ→Math! :p":bool
  in  "selection :|\\":u16(ring)=6 caption="files" items=["IDS063_210603_RAW_cal_Indium_2nd_063_C(f)_35.0T_0.8K_0deg_Tdep_dc_bias_raw_.dat", "IDS008_210601_RAW_cal_Indium_2nd_008_C(f)_35.0T_1.0K_0deg_Bdep_raw_.dat", "IDS013_210601_RAW_cal_Indium_2nd_013_C(f)_35.0T_1.0K_0deg_Bdep_raw_.dat", "IDS061_210603_RAW_cal_Indium_2nd_061_C(f)_35.0T_1.0K_0deg_Tdep_dc_bias_raw_.dat", "IDS076_210604_RAW_cal_Indium_2nd_076_C(f)_35.0T_1.2K_0deg_Tdep_dc_bias_raw_.dat", "IDS064_210603_RAW_cal_Indium_2nd_064_C(f)_35.0T_1.38K_0deg_Tdep_dc_bias_raw_.dat", "IDS075_210604_RAW_cal_Indium_2nd_075_C(f)_35.0T_1.6K_0deg_Tdep_dc_bias_raw_.dat", "IDS065_210603_RAW_cal_Indium_2nd_065_C(f)_35.0T_1.83K_0deg_Tdep_dc_bias_raw_.dat", "IDS074_210604_RAW_cal_Indium_2nd_074_C(f)_35.0T_2.13K_0deg_Tdep_dc_bias_raw_.dat", "IDS066_210603_RAW_cal_Indium_2nd_066_C(f)_35.0T_2.55K_0deg_Tdep_dc_bias_raw_.dat", "IDS019_210602_RAW_cal_Indium_2nd_019_C(f)_35.0T_3.0K_0deg_Tdep_raw_.dat", "IDS069_210604_RAW_cal_Indium_2nd_069_C(f)_35.0T_4.0K_0deg_Tdep_dc_bias_raw_.dat", "IDS067_210603_RAW_cal_Indium_2nd_067_C(f)_35.0T_8.2K_0deg_Tdep_dc_bias_raw_.dat"]
  in  "tab 5":enum32{"Page 1"}(tab)
  in  "Math→τ! :q":bool
  in  "tab 44":enum32{"default values "}(tab)
  in  "defaults selector":T9(array[cluster])=[{"Plost: sweep window"=enum."ζ", "used default"=FALSE}, {"Plost: sweep window"=enum."τ1", "used default"=FALSE}, {"Plost: sweep window"=enum."τS", "used default"=FALSE}, {"Plost: sweep window"=enum."τN", "used default"=FALSE}, {"Plost: sweep window"=enum."τC", "used default"=FALSE}, {"Plost: sweep window"=enum."κ0", "used default"=FALSE}]
  in  "default values string":string="\"0\"->   <|\"T\" -> 0.120000, \"τN\"-> 0.670097, \"τC\"-> 0.003, \"ζ\"-> 0.368640, \"κ0\"-> 0.00000000044100|>   ,\n\"1\"->   <|\"T\" -> 0.220000, \"τN\"-> 0.057428, \"τC\"-> 0.001386, \"ζ\"-> 0.131633, \"κ0\"-> 0.00000000120283|>   ,\n\"2\"->   <|\"T\" -> 0.320000, \"τN\"-> 0.014576, \"τC\"-> 0.001971, \"ζ\"-> 0.063259, \"κ0\"-> 0.00000000186767|>   ,\n\"3\"->   <|\"T\" -> 0.420000, \"τN\"-> 0.005816, \"τC\"-> 0.002645, \"ζ\"-> 0.041943, \"κ0\"-> 0.00000000259214|>   ,\n\"4\"->   <|\"T\" -> 0.520000, \"τN\"-> 0.002807, \"τC\"-> 0.003188, \"ζ\"-> 0.030182, \"κ0\"-> 0.00000000339327|>   ,\n\"5\"->   <|\"T\" -> 0.620000, \"τN\"-> 0.001928, \"τC\"-> 0.003634, \"ζ\"-> 0.025126, \"κ0\"-> 0.00000000404950|>   ,\n\"6\"->   <|\"T\" -> 0.720000, \"τN\"-> 0.001251, \"τC\"-> 0.004021, \"ζ\"-> 0.023386, \"κ0\"-> 0.00000000484450|>   ,\n\"7\"->   <|\"T\" -> 0.820000, \"τN\"-> 0.000866, \"τC\"-> 0.004389, \"ζ\"-> 0.022054, \"κ0\"-> 0.00000000563624|>   ,\n\"8\"->   <|\"T\" -> 0.920000, \"τN\"-> 0.000673, \"τC\"-> 0.004723, \"ζ\"-> 0.021623, \"κ0\"-> 0.00000000639866|>   ,\n\"9\"->   <|\"T\" -> 1.020000, \"τN\"-> 0.000537, \"τC\"-> 0.005044, \"ζ\"-> 0.021243, \"κ0\"-> 0.00000000716107|>   ,\n\"10\"->   <|\"T\" -> 1.120000, \"τN\"-> 0.000431, \"τC\"-> 0.005344, \"ζ\"-> 0.020967, \"κ0\"-> 0.00000000793323|>   ,\n\"11\"->   <|\"T\" -> 1.220000, \"τN\"-> 0.000336, \"τC\"-> 0.005596, \"ζ\"-> 0.020955, \"κ0\"-> 0.00000000874437|>   ,\n\"12\"->   <|\"T\" -> 1.320000, \"τN\"-> 0.000267, \"τC\"-> 0.005838, \"ζ\"-> 0.020944, \"κ0\"-> 0.00000000955551|>   ,\n\"13\"->   <|\"T\" -> 1.420000, \"τN\"-> 0.000216, \"τC\"-> 0.006071, \"ζ\"-> 0.020934, \"κ0\"-> 0.00000001036666|>   ,\n\"14\"->   <|\"T\" -> 1.520000, \"τN\"-> 0.000177, \"τC\"-> 0.006297, \"ζ\"-> 0.020925, \"κ0\"-> 0.00000001117780|>   ,\n\"15\"->   <|\"T\" -> 1.620000, \"τN\"-> 0.000147, \"τC\"-> 0.006517, \"ζ\"-> 0.020916, \"κ0\"-> 0.00000001198894|>   ,\n\"16\"->   <|\"T\" -> 1.720000, \"τN\"-> 0.000123, \"τC\"-> 0.006730, \"ζ\"-> 0.020907, \"κ0\"-> 0.00000001280009|>   ,\n\"17\"->   <|\"T\" -> 1.820000, \"τN\"-> 0.000105, \"τC\"-> 0.006885, \"ζ\"-> 0.020876, \"κ0\"-> 0.00000001362415|>   ,\n\"18\"->   <|\"T\" -> 1.920000, \"τN\"-> 0.000091, \"τC\"-> 0.006831, \"ζ\"-> 0.020754, \"κ0\"-> 0.00000001449990|>   ,\n\"19\"->   <|\"T\" -> 2.020000, \"τN\"-> 0.000080, \"τC\"-> 0.006781, \"ζ\"-> 0.020639, \"κ0\"-> 0.00000001537565|>   ,\n\"20\"->   <|\"T\" -> 2.120000, \"τN\"-> 0.000070, \"τC\"-> 0.006733, \"ζ\"-> 0.020530, \"κ0\"-> 0.00000001625140|>   ,\n\"21\"->   <|\"T\" -> 2.220000, \"τN\"-> 0.000062, \"τC\"-> 0.006687, \"ζ\"-> 0.020427, \"κ0\"-> 0.00000001712715|>   ,\n\"22\"->   <|\"T\" -> 2.320000, \"τN\"-> 0.000056, \"τC\"-> 0.006644, \"ζ\"-> 0.020329, \"κ0\"-> 0.00000001800290|>   ,\n\"23\"->   <|\"T\" -> 2.420000, \"τN\"-> 0.000050, \"τC\"-> 0.006603, \"ζ\"-> 0.020235, \"κ0\"-> 0.00000001887865|>   ,\n\"24\"->   <|\"T\" -> 2.520000, \"τN\"-> 0.000045, \"τC\"-> 0.006564, \"ζ\"-> 0.020146, \"κ0\"-> 0.00000001975440|>   ,\n\"25\"->   <|\"T\" -> 2.620000, \"τN\"-> 0.000040, \"τC\"-> 0.006527, \"ζ\"-> 0.020060, \"κ0\"-> 0.00000002063015|>   ,\n\"26\"->   <|\"T\" -> 2.720000, \"τN\"-> 0.000037, \"τC\"-> 0.006491, \"ζ\"-> 0.019978, \"κ0\"-> 0.00000002150590|>   ,\n\"27\"->   <|\"T\" -> 2.820000, \"τN\"-> 0.000033, \"τC\"-> 0.006457, \"ζ\"-> 0.019899, \"κ0\"-> 0.00000002238165|>   ,\n\"28\"->   <|\"T\" -> 2.920000, \"τN\"-> 0.000030, \"τC\"-> 0.006424, \"ζ\"-> 0.019824, \"κ0\"-> 0.00000002325740|>   ,\n\"29\"->   <|\"T\" -> 3.020000, \"τN\"-> 0.000028, \"τC\"-> 0.006374, \"ζ\"-> 0.019852, \"κ0\"-> 0.00000002421662|>   ,\n\"30\"->   <|\"T\" -> 3.120000, \"τN\"-> 0.000026, \"τC\"-> 0.006255, \"ζ\"-> 0.020282, \"κ0\"-> 0.00000002550973|>   ,\n\"31\"->   <|\"T\" -> 3.220000, \"τN\"-> 0.000024, \"τC\"-> 0.006143, \"ζ\"-> 0.020708, \"κ0\"-> 0.00000002680284|>   ,\n\"32\"->   <|\"T\" -> 3.320000, \"τN\"-> 0.000023, \"τC\"-> 0.006036, \"ζ\"-> 0.021130, \"κ0\"-> 0.00000002809596|>   ,\n\"33\"->   <|\"T\" -> 3.420000, \"τN\"-> 0.000021, \"τC\"-> 0.005933, \"ζ\"-> 0.021547, \"κ0\"-> 0.00000002938907|>   ,\n\"34\"->   <|\"T\" -> 3.520000, \"τN\"-> 0.000020, \"τC\"-> 0.005836, \"ζ\"-> 0.021960, \"κ0\"-> 0.00000003068218|>   ,\n\"35\"->   <|\"T\" -> 3.620000, \"τN\"-> 0.000019, \"τC\"-> 0.005742, \"ζ\"-> 0.022368, \"κ0\"-> 0.00000003197529|>   ,\n\"36\"->   <|\"T\" -> 3.720000, \"τN\"-> 0.000018, \"τC\"-> 0.005653, \"ζ\"-> 0.022774, \"κ0\"-> 0.00000003326840|>   ,\n\"37\"->   <|\"T\" -> 3.820000, \"τN\"-> 0.000017, \"τC\"-> 0.005567, \"ζ\"-> 0.023175, \"κ0\"-> 0.00000003456151|>   ,\n\"38\"->   <|\"T\" -> 3.920000, \"τN\"-> 0.000016, \"τC\"-> 0.005485, \"ζ\"-> 0.023573, \"κ0\"-> 0.00000003585462|>   ,\n\"39\"->   <|\"T\" -> 4.020000, \"τN\"-> 0.000015, \"τC\"-> 0.005406, \"ζ\"-> 0.023967, \"κ0\"-> 0.00000003714773|>   ,\n\"40\"->   <|\"T\" -> 4.120000, \"τN\"-> 0.000014, \"τC\"-> 0.005330, \"ζ\"-> 0.024358, \"κ0\"-> 0.00000003844084|>   ,\n\"41\"->   <|\"T\" -> 4.220000, \"τN\"-> 0.000013, \"τC\"-> 0.005257, \"ζ\"-> 0.024746, \"κ0\"-> 0.00000003973396|>   ,\n\"42\"->   <|\"T\" -> 4.320000, \"τN\"-> 0.000013, \"τC\"-> 0.005186, \"ζ\"-> 0.025131, \"κ0\"-> 0.00000004102707|>   ,\n\"43\"->   <|\"T\" -> 4.420000, \"τN\"-> 0.000012, \"τC\"-> 0.005118, \"ζ\"-> 0.025512, \"κ0\"-> 0.00000004232018|>   ,\n\"44\"->   <|\"T\" -> 4.520000, \"τN\"-> 0.000012, \"τC\"-> 0.005053, \"ζ\"-> 0.025891, \"κ0\"-> 0.00000004361329|>   ,\n\"45\"->   <|\"T\" -> 4.620000, \"τN\"-> 0.000011, \"τC\"-> 0.004990, \"ζ\"-> 0.026267, \"κ0\"-> 0.00000004490640|>   ,\n\"46\"->   <|\"T\" -> 4.720000, \"τN\"-> 0.000011, \"τC\"-> 0.004928, \"ζ\"-> 0.026640, \"κ0\"-> 0.00000004619951|>   ,\n\"47\"->   <|\"T\" -> 4.820000, \"τN\"-> 0.000010, \"τC\"-> 0.004869, \"ζ\"-> 0.027010, \"κ0\"-> 0.00000004749262|>   ,\n\"48\"->   <|\"T\" -> 4.920000, \"τN\"-> 0.000010, \"τC\"-> 0.004812, \"ζ\"-> 0.027378, \"κ0\"-> 0.00000004878573|>   ,"
  in  "load default values":bool
  in  "selector":T10={"ignore set of !"=TRUE, "set (1T|2B)"=0, "ignore side !"=FALSE, "side (8S|4R)"=0, "ignore θ !"=FALSE, "ignore B !"=FALSE, "T (K)"=1, "ignore T !"=TRUE, "θ (deg)"=0, "B (T)"=5, "lookup"={"set of lookup"={0=1.0, 1=2.0}, "all set of"={1.0, 2.0}, "T lookup"={0=0.12, 1=0.122, 2=0.14, 3=0.148, 4=0.15, 5=0.157, 6=0.16, 7=0.168, 8=0.17, 9=0.178, 10=0.179, 11=0.19, 12=0.197, 13=0.2, 14=0.22, 15=0.249, 16=0.25, 17=0.255, 18=0.26, 19=0.28, 20=0.3, 21=0.307, 22=0.308, 23=0.31, 24=0.33, 25=0.36, 26=0.4, 27=0.42, 28=0.43, 29=0.438, 30=0.48, 31=0.512, 32=0.52, 33=0.53, 34=0.58, 35=0.61, 36=0.62, 37=0.63, 38=0.677, 39=0.68, 40=0.81, 41=0.82, 42=0.83, 43=0.91, 44=1.0, 45=1.1, 46=1.12, 47=1.13, 48=1.23, 49=1.25, 50=1.28, 51=1.31, 52=1.39, 53=1.52, 54=1.55, 55=1.7, 56=1.8, 57=1.9, 58=1.97, 59=2.1, 60=2.3, 61=3.0, 62=3.07, 63=3.1, 64=3.11, 65=3.19, 66=5.7, 67=5.75, 68=5.8}, "θ lookup"={0=0.0, 1=30.0, 2=45.0, 3=60.0, 4=90.0}, "B lookup"={0=0.0, 1=1.0, 2=2.0, 3=4.0, 4=5.0, 5=6.0, 6=7.0, 7=8.0, 8=9.0, 9=10.0, 10=11.0, 11=12.0}, "all T's"={0.12, 0.122, 0.14, 0.148, 0.15, 0.157, 0.16, 0.168, 0.17, 0.178, 0.179, 0.19, 0.197, 0.2, 0.22, 0.249, 0.25, 0.255, 0.26, 0.28, 0.3, 0.307, 0.308, 0.31, 0.33, 0.36, 0.4, 0.42, 0.43, 0.438, 0.48, 0.512, 0.52, 0.53, 0.58, 0.61, 0.62, 0.63, 0.677, 0.68, 0.81, 0.82, 0.83, 0.91, 1.0, 1.1, 1.12, 1.13, 1.23, 1.25, 1.28, 1.31, 1.39, 1.52, 1.55, 1.7, 1.8, 1.9, 1.97, 2.1, 2.3, 3.0, 3.07, 3.1, 3.11, 3.19, 5.7, 5.75, 5.8}, "all θ's"={0.0, 30.0, 45.0, 60.0, 90.0}, "all B's"={0.0, 1.0, 2.0, 4.0, 5.0, 6.0, 7.0, 8.0, 9.0, 10.0, 11.0, 12.0}, "all sides"={4000.0, 8000.0}, "side lookup"={0=4000.0, 1=8000.0}}} {"B (T)" items=["0.000", "5.000", "10.000", "15.000", "20.000", "25.000", "30.000", "35.000"]; "θ (deg)" items=["0.000"]; "T (K)" items=["0.800", "1.000", "1.200", "1.380", "1.400", "1.600", "1.800", "1.830", "2.130", "2.550", "2.560", "3.000", "4.000", "5.000", "8.200"]; "side (8S|4R)" items=["4000", "8000"]; "set (1T|2B)" items=["1", "2"]}
  in  "parameter selectors tab":enum32{"Page 1"}(tab)
  in  "colors":u32[](array[colorbox])=[7087058, 56538, 2062078, 16740827, 16755712, 11121611, 8285330, 9272482, 9204890]
  in  "parameter":T2[](array[typedef])=[enum."ζ", enum."τ1", enum."τS", enum."τN", enum."τC", enum."κ0"]
  in  "curvature & stuff":enum32{"Page 2", "Page 1", "Page 3"}(tab)=enum."Page 1"
  in  "error goodness weighting":T5
  in  "sampling size(%)":dbl(slide)=0.01 scale=0.001..1.0 scale format="%#_2p"
  in  "curvature triplets":T11[](array[typedef])=[{"one"=enum."τ1", "two"=enum."τS", "sigmaone"=enum."στ1", "sigmatwo"=enum."στS", "3D curvature"={"curvature Matrix"=[[0.4507078460882445, -2.1760838828759383, -1.280990861794483], [-2.1760838828759383, 322.0085679089189, 2.353318922157897], [-1.280990861794483, 2.353318922157897, 0.6755839942885177]], "eigenvs"=[322.0406532275578, -0.7227707615937441, 1.8169772833316062], "Eigenvectors"=[[-0.8506508083520399+0.0i, -0.5257311121191335+0.0i], [0.5257311121191335+0.0i, -0.8506508083520399+0.0i]], "theta (rad)"=0.5746565280690623, "theta (deg)"=32.9253937279984, "Δs"=[0.032347659490051216, 0.00010225804136915292, 0.0011727018719404464], "δG/G"=0.5535743588970453, "Δlog(s)"=[0.07080165473171017, 0.005621411995797319, 0.05761660609327092], "inverse Matrix"=[[-0.5012874312748296, 0.0036518573945886344, -0.9632238318323554], [0.0036518573945884536, 0.0031600272826493997, -0.004083216996066563], [-0.963223831832355, -0.0040832169960665216, -0.33196732977071436]], "noise T"=0.1}, "three"=enum."τN", "sigmathree"=enum."στN", "pars & errors"={}}] {"3D curvature"."noise T" format="%#_3f"; "3D curvature"."inverse Matrix" format="%#_3p"; "3D curvature"."Δlog(s)" scale=0.001..10.0; "3D curvature"."δG/G" format="%#_3f"; "3D curvature"."Δs" format="%#_2p"; "3D curvature"."theta (deg)" format="%#_3p"; "3D curvature"."curvature Matrix" format="%#_3p"; "3D curvature"."eigenvs" format="%#_2f"; "3D curvature"."Eigenvectors" format="%#_3p"; "3D curvature"."theta (rad)" format="%#_3p"}
  in  "update  as you fit":bool=TRUE
  in  "error-mode":T15
  in  "tab 10":enum32{"Page 1"}(tab)
  in  "hist size":i32=300
  out "Plot: curvature":cluster{"Freq out (Hz)":dbl[], dbl[]}[](graph)
  in  "scale gauge: Plot: curvatures":dbl(slide)=4.2999999999999995e-05 min=0.0 max=0.3 step=1e-06 scale=1e-09..1.0 scale format="%#_3p"
  in  "ω0 (rad/sec)":dbl(slide)=19.063235402868393 scale=0.001..50000.0 scale format="%#_2p"
  in  "load & stuff tab":enum32{"Page 2"}(tab)
  in  "|ω| < limit (Hz)":dbl(slide)=1040.0 min=10.0 max=10000.0 step=10.0 scale=50.0..5000.0 scale format="%#_3p"
  in  "offset Re\noffset Im":cluster{"Numeric":dbl, "Numeric":dbl}(slide)={"Numeric"=-461224.48979591834, "Numeric"=0.0} scale=-1000000.0..10000000.0 scale format="%#_1p"
  in  "overwrite offset":bool=TRUE
  in  "filenames":u16(ring)=29 caption="files" items=["IDS034_210602_RAW_cal_Indium_2nd_034_C(f)_25.0T_0.8K_0deg_Tdep_raw_.dat", "IDS036_210602_RAW_cal_Indium_2nd_036_C(f)_30.0T_0.8K_0deg_Tdep_raw_.dat", "IDS037_210602_RAW_cal_Indium_2nd_037_C(f)_15.0T_0.8K_0deg_Tdep_raw_.dat", "IDS038_210602_RAW_cal_Indium_2nd_038_C(f)_0.0T_0.8K_0deg_Tdep_raw_.dat", "IDS063_210603_RAW_cal_Indium_2nd_063_C(f)_35.0T_0.8K_0deg_Tdep_dc_bias_raw_.dat", "IDS008_210601_RAW_cal_Indium_2nd_008_C(f)_35.0T_1.0K_0deg_Bdep_raw_.dat", "IDS009_210601_RAW_cal_Indium_2nd_009_C(f)_25.0T_1.0K_0deg_Bdep_raw_.dat", "IDS010_210601_RAW_cal_Indium_2nd_010_C(f)_10.0T_1.0K_0deg_Bdep_raw_.dat", "IDS011_210601_RAW_cal_Indium_2nd_011_C(f)_20.0T_1.0K_0deg_Bdep_raw_.dat", "IDS012_210601_RAW_cal_Indium_2nd_012_C(f)_30.0T_1.0K_0deg_Bdep_raw_.dat", "IDS013_210601_RAW_cal_Indium_2nd_013_C(f)_35.0T_1.0K_0deg_Bdep_raw_.dat", "IDS014_210601_RAW_cal_Indium_2nd_014_C(f)_15.0T_1.0K_0deg_Bdep_raw_.dat", "IDS015_210601_RAW_cal_Indium_2nd_015_C(f)_5.0T_1.0K_0deg_Bdep_raw_.dat", "IDS016_210601_RAW_cal_Indium_2nd_016_C(f)_0.0T_1.0K_0deg_Bdep_raw_.dat", "IDS053_210603_RAW_cal_Indium_2nd_053_C(f)_0.0T_1.0K_0deg_Tdep_dc_bias_raw_.dat", "IDS055_210603_RAW_cal_Indium_2nd_055_C(f)_5.0T_1.0K_0deg_Tdep_dc_bias_raw_.dat", "IDS057_210603_RAW_cal_Indium_2nd_057_C(f)_15.0T_1.0K_0deg_Tdep_dc_bias_raw_.dat", "IDS058_210603_RAW_cal_Indium_2nd_058_C(f)_20.0T_1.0K_0deg_Tdep_dc_bias_raw_.dat", "IDS059_210603_RAW_cal_Indium_2nd_059_C(f)_25.0T_1.0K_0deg_Tdep_dc_bias_raw_.dat", "IDS060_210603_RAW_cal_Indium_2nd_060_C(f)_30.0T_1.0K_0deg_Tdep_dc_bias_raw_.dat", "IDS061_210603_RAW_cal_Indium_2nd_061_C(f)_35.0T_1.0K_0deg_Tdep_dc_bias_raw_.dat", "IDS062_210603_RAW_cal_Indium_2nd_062_C(f)_10.0T_1.0K_0deg_Tdep_dc_bias_raw_.dat", "IDS043_210603_RAW_cal_Indium_2nd_043_C(f)_15.0T_1.2K_0deg_Tdep_raw_.dat", "IDS044_210603_RAW_cal_Indium_2nd_044_C(f)_25.0T_1.2K_0deg_Tdep_raw_.dat", "IDS045_210603_RAW_cal_Indium_2nd_045_C(f)_30.0T_1.2K_0deg_Tdep_raw_.dat", "IDS049_210603_RAW_cal_Indium_2nd_049_C(f)_0.0T_1.2K_0deg_Tdep_raw_.dat", "IDS050_210603_RAW_cal_Indium_2nd_050_C(f)_0.0T_1.2K_0deg_Tdep_raw_.dat", "IDS051_210603_RAW_cal_Indium_2nd_051_C(f)_0.0T_1.2K_0deg_Tdep_raw_.dat", "IDS052_210603_RAW_cal_Indium_2nd_052_C(f)_0.0T_1.2K_0deg_Tdep_dc_bias_raw_.dat", "IDS076_210604_RAW_cal_Indium_2nd_076_C(f)_35.0T_1.2K_0deg_Tdep_dc_bias_raw_.dat", "IDS064_210603_RAW_cal_Indium_2nd_064_C(f)_35.0T_1.38K_0deg_Tdep_dc_bias_raw_.dat", "IDS030_210602_RAW_cal_Indium_2nd_030_C(f)_15.0T_1.4K_0deg_Tdep_raw_.dat", "IDS032_210602_RAW_cal_Indium_2nd_032_C(f)_30.0T_1.4K_0deg_Tdep_raw_.dat", "IDS033_210602_RAW_cal_Indium_2nd_033_C(f)_25.0T_1.4K_0deg_Tdep_raw_.dat", "IDS039_210602_RAW_cal_Indium_2nd_039_C(f)_0.0T_1.4K_0deg_Tdep_raw_.dat", "IDS027_210602_RAW_cal_Indium_2nd_027_C(f)_30.0T_1.6K_0deg_Tdep_raw_.dat", "IDS028_210602_RAW_cal_Indium_2nd_028_C(f)_25.0T_1.6K_0deg_Tdep_raw_.dat", "IDS029_210602_RAW_cal_Indium_2nd_029_C(f)_15.0T_1.6K_0deg_Tdep_raw_.dat", "IDS040_210602_RAW_cal_Indium_2nd_040_C(f)_0.0T_1.6K_0deg_Tdep_raw_.dat", "IDS075_210604_RAW_cal_Indium_2nd_075_C(f)_35.0T_1.6K_0deg_Tdep_dc_bias_raw_.dat", "IDS024_210602_RAW_cal_Indium_2nd_024_C(f)_25.0T_1.8K_0deg_Tdep_raw_.dat", "IDS025_210602_RAW_cal_Indium_2nd_025_C(f)_15.0T_1.8K_0deg_Tdep_raw_.dat", "IDS026_210602_RAW_cal_Indium_2nd_026_C(f)_30.0T_1.8K_0deg_Tdep_raw_.dat", "IDS041_210602_RAW_cal_Indium_2nd_041_C(f)_0.0T_1.8K_0deg_Tdep_raw_.dat", "IDS065_210603_RAW_cal_Indium_2nd_065_C(f)_35.0T_1.83K_0deg_Tdep_dc_bias_raw_.dat", "IDS074_210604_RAW_cal_Indium_2nd_074_C(f)_35.0T_2.13K_0deg_Tdep_dc_bias_raw_.dat", "IDS066_210603_RAW_cal_Indium_2nd_066_C(f)_35.0T_2.55K_0deg_Tdep_dc_bias_raw_.dat", "IDS081_210604_RAW_cal_Indium_2nd_081_C(f)_25.0T_2.56K_0deg_Tdep_dc_bias_raw_.dat", "IDS019_210602_RAW_cal_Indium_2nd_019_C(f)_35.0T_3.0K_0deg_Tdep_raw_.dat", "IDS080_210604_RAW_cal_Indium_2nd_080_C(f)_25.0T_3.0K_0deg_Tdep_dc_bias_raw_.dat", "IDS069_210604_RAW_cal_Indium_2nd_069_C(f)_35.0T_4.0K_0deg_Tdep_dc_bias_raw_.dat", "IDS070_210604_RAW_cal_Indium_2nd_070_C(f)_15.0T_4.0K_0deg_Tdep_dc_bias_raw_.dat", "IDS042_210602_RAW_cal_Indium_2nd_042_C(f)_0.0T_5.0K_0deg_Tdep_raw_.dat", "IDS067_210603_RAW_cal_Indium_2nd_067_C(f)_35.0T_8.2K_0deg_Tdep_dc_bias_raw_.dat", "IDS068_210603_RAW_cal_Indium_2nd_068_C(f)_25.0T_8.2K_0deg_Tdep_dc_bias_raw_.dat"]
  in  "folder":path=path "/opt/new/Dropbox/shared_AkashAndreas/paper-CeCoIn5/Original RAW data"
  in  "file pattern":string="IDS*RAW*_raw_.dat"
  in  "string IN → Math!":bool
  in  "Math→ string OUT! :s":bool
